vi "ST5520_TEST_OP150.vi"(6 "Application Directory":path caption="Répertoire de l'application", 7 "key 2":string, 8 "errin":errorcluster, 9 "key":string, 10 "lbl log std":string, 11 "ST5520":refnum<visa-resource-name>) -> (0 "errout":errorcluster, 1 "R iso(MOhm)":dbl, 2 "LOG STD":string, 3 "OK?":bool, 4 "dbl":dbl, 5 "sous-chaîne précédente":string)   [LabVIEW 2020]
panel:
  out "dbl 2":dbl
  out "x = y ?":bool
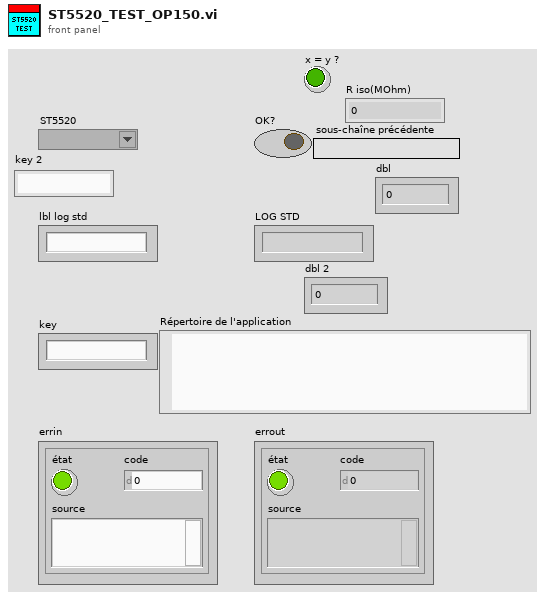
[diagram p1: front panel]
types:
  T1 = enum16{"Normal", "Over Flow", "Under Flow", "Error"}
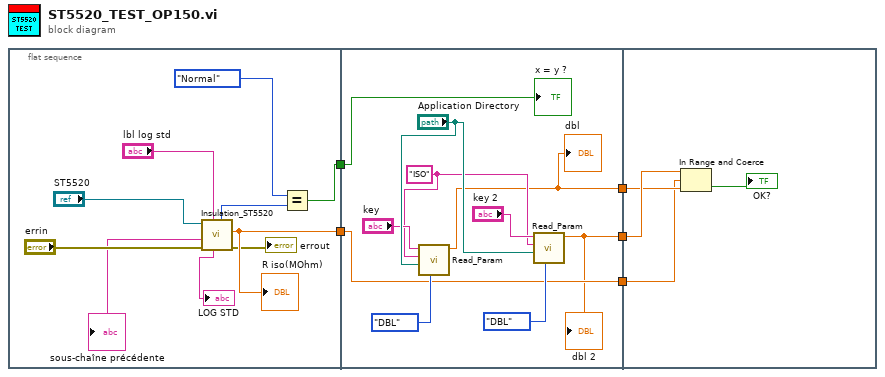
[diagram p0: block diagram]
diagram:
  n1 = flat-sequence {
    tunnel: [w15] -> w5
    tunnel: [w8] -> w4
    tunnel: w5 -> [w22]
    tunnel: w4 -> [w18]
    tunnel: [w16] -> w3
    tunnel: [w17] -> w2
    tunnel: [w18] -> w1
    tunnel: w3 -> [w28]
    tunnel: w2 -> [w27]
    tunnel: w1 -> [w26]
    frame #0 {
      n2 = call <userlib>:"Insulation_ST5520.vi"("lbl log std"="lbl log std", "errin"="errin", "Refnum VISA en entrée"="ST5520") -> ("error out"=→"errout":errorcluster, "R iso(MOhm)"=w8:dbl, "Status"=w13:T1, "LOG STD"=→"LOG STD":string, "sous-chaîne précédente"=→"sous-chaîne précédente":string)  [unwired: 4 out]
      "R iso(MOhm)" <- w8
      n3 = Equal?(x=T1."Normal" ("Status"), y=w13) -> (x = y?=w15:bool)
    }
    frame #1 {
      w20 = "ISO" ("section")
      n4 = call <userlib>:"Read_Param.vi"("Énum"=enum16{"STR", "DBL", "U32", "chemin"}."DBL", "pathin"="Application Directory", "section"=w20, "key"="key") -> ("dbl"=w17:dbl)  [unwired: 3 in, 4 out]
      "dbl" <- w17
      n5 = call <userlib>:"Read_Param.vi"("Énum"=enum16{"STR", "DBL", "U32", "chemin"}."DBL", "pathin"="Application Directory", "section"=w20, "key"="key 2") -> ("dbl"=w16:dbl)  [unwired: 3 in, 4 out]
      "dbl 2" <- w16
      "x = y ?" <- w22
    }
    frame #2 {
      n6 = In Range and Coerce(upper limit=w28, x=w26, lower limit=w27) -> (In Range?=→"OK?":bool)  [unwired: 1 out]
    }
  }
